vi "MOV_Z_core_colse.vi"(1 "error in (no error)":errorcluster, 2 "VISA resource name":refnum<visa-resource-name>) -> ()   [LabVIEW 2013]
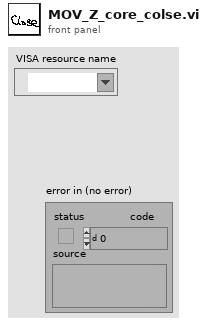
[diagram p1: front panel]
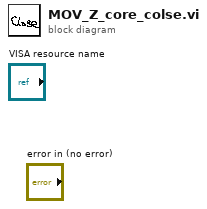
[diagram p0: block diagram]
diagram:
